vi "Decimate (single).vi"(8 "error in (no error)":errorcluster, 9 "averaging (off)":bool, 10 "decimating factor (1)":i32=1, 11 "XY-data":cluster{"X-array":dbl[], "Y-array":dbl[]}) -> (0 "error out":errorcluster, 3 "XY-data out":cluster{"X-array":dbl[], "Y-array":dbl[]} {"Y-array" format="%.2p"; "X-array" format="%.2p"})   [LabVIEW 2016, in "xy_utilities.lvlib"]
doc: "Decimates the input <b>XY-data</b> by the <b>decimating factor</b> and the <b>averaging</b> Boolean control. \n\nWire data to the data input to determine the polymorphic instance to use or manually select the instance."
uses:
  xy_utilities.lvlib
  <vilib>/Analysis/2dsp.llb/Decimate (single shot, DBL).vi
  <vilib>/Analysis/NI_AALPro.lvlib
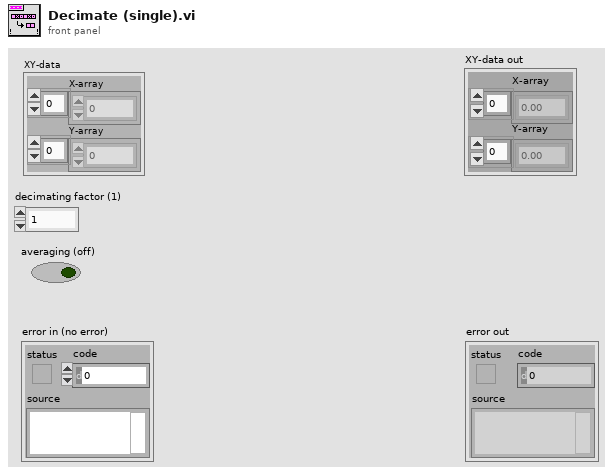
[diagram p1: front panel]
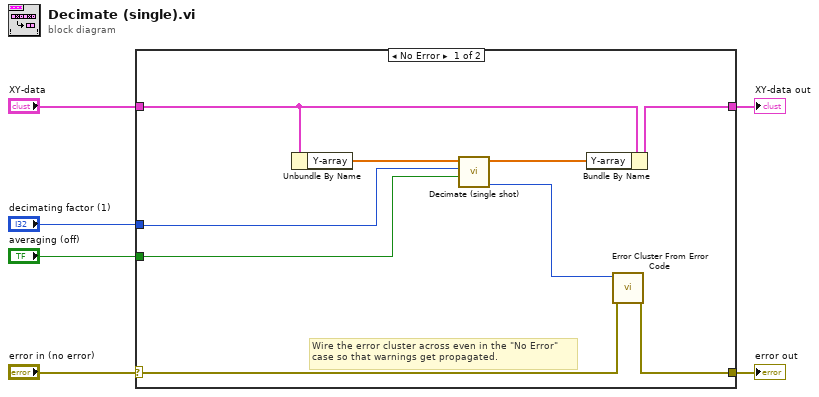
[diagram p0: block diagram]
diagram:
  n1 = case shown="No Error" "error in (no error)" {
    selector: "error in (no error)" -> [w10 w17]
    tunnel: [w9 w17] -> w5
    tunnel: "XY-data" -> [w15 w16]
    tunnel: [w14 w16] -> w3
    tunnel: "decimating factor (1)" -> [w8 _]
    tunnel: "averaging (off)" -> [w7 _]
    frame No Error {
      # "Wire the error cluster across even in the \"No Error\"\ncase so that warnings get propagated."
      n2 = Unbundle By Name(w15) -> ("Y-array"=w13:dbl[])
      n3 = call-poly <vilib>:"Decimate (single shot).vi"("averaging"=w7, "decimating factor"=w8, "X"=w13) -> ("error"=w11:i32, "Decimated Array"=w12:dbl[])  [unwired: 7 in]
      n4 = Bundle By Name(cluster=w15, "Y-array"=w12) -> (w14:cluster{"X-array":dbl[], "Y-array":dbl[]})
      n5 = call <vilib>:"Error Cluster From Error Code.vi"("error in (no error)"=w10, "error code (0)"=w11) -> ("error out"=w9:errorcluster)  [unwired: 7 in]
    }
    frame Error {
    }
  }
  "error out" <- w5
  "XY-data out" <- w3
